vi "send_ThrottleSteeringRaw.vi"(4 "Counter":i32, 5 "200/freq":i32=1, 6 "Active":bool, 7 "CAN ID":u32=512 format="%x", 8 "Message":T2 {"APPS2" scale=0.0..4095.0; "APPS1" scale=0.0..4095.0; "Steering Angle 2" scale=0.0..4095.0; "Steering Angle 1" scale=0.0..4095.0}, 11 "CAN frame":T1[](array[typedef]) {"Data" format="%.0x"; "ArbitrationId" format="%.0x"; "Timestamp" format="%<%I:%M:%S%3u %p\n%m/%d/%Y>T"}) -> (3 "CAN frame out":T1[](array[typedef]) {"Data" format="%.0x"; "ArbitrationId" format="%.0x"; "Timestamp" format="%<%I:%M:%S%3u %p\n%m/%d/%Y>T"})   [LabVIEW 2017]
uses:
  <vilib>/nican/nican.llb/CanFrameTimed.ctl
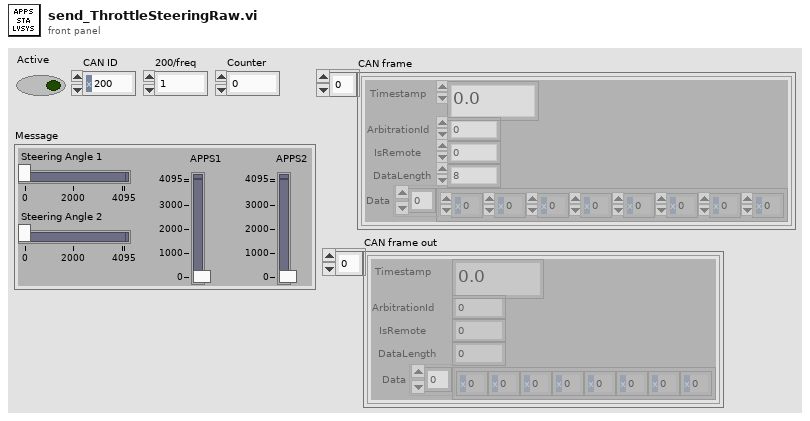
[diagram p1: front panel]
types:
  T1 = typedef "CanFrameTimed.ctl" = cluster{"Timestamp":dbl, "ArbitrationId":u32, "IsRemote":u8, "DataLength":u8, "Data":u8[]}
  T2 = cluster{"Steering Angle 1":u16, "Steering Angle 2":u16, "APPS1":u16, "APPS2":u16}
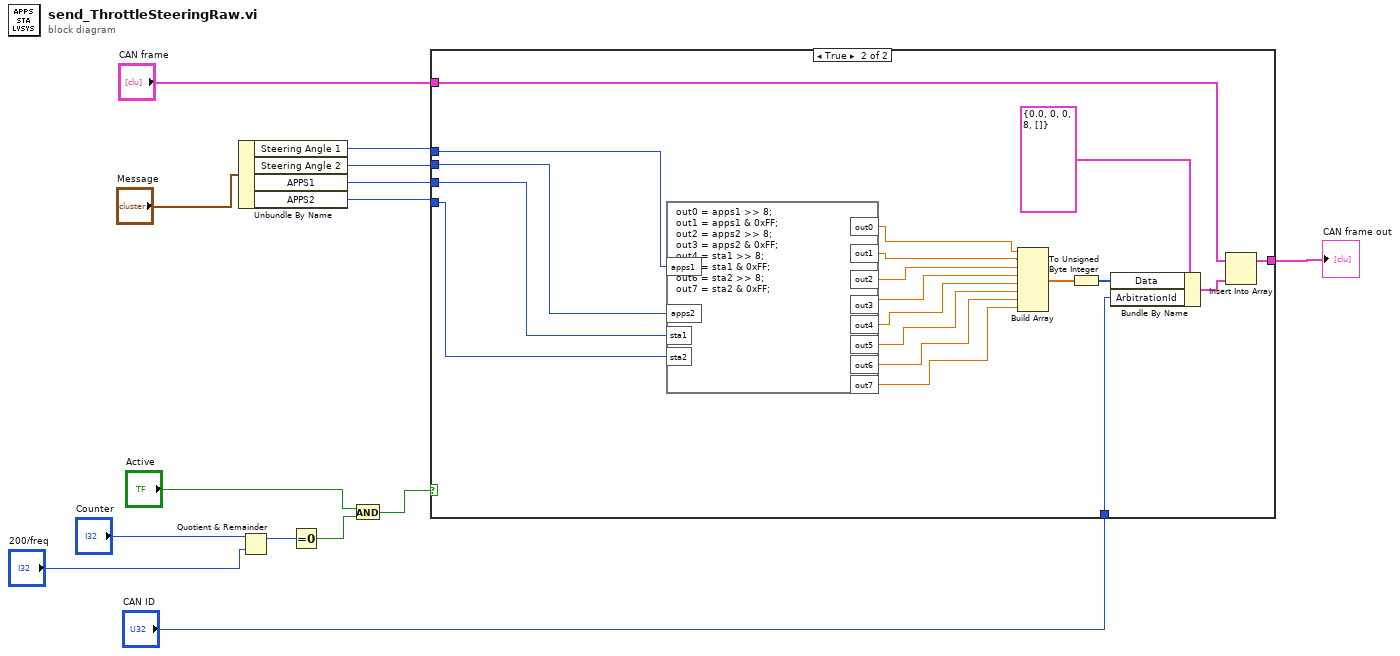
[diagram p0: block diagram]
diagram:
  n1 = Unbundle By Name("Message") -> ("Steering Angle 1"=w12:u16, "Steering Angle 2"=w13:u16, "APPS1"=w11:u16, "APPS2"=w10:u16)
  n2 = Quotient & Remainder(x="Counter", y="200/freq") -> (x-y*floor(x/y)=w5:i32)  [unwired: 1 out]
  n3 = Equal To 0?(x=w5) -> (x = 0?=w3:bool)
  n4 = And(x="Active", y=w3) -> (x .and. y?=w2:bool)
  n5 = case shown="True" w2 {
    tunnel: w13 -> [_ w18]
    tunnel: w12 -> [_ w19]
    tunnel: w11 -> [_ w17]
    tunnel: w10 -> [_ w16]
    tunnel: "CAN frame" -> [w15 w23]
    tunnel: [w15 w21] -> w8
    tunnel: "CAN ID" -> [_ w20]
    frame False {
    }
    frame True {
      n6 = formula code="out0 = apps1 >> 8;\nout1 = apps1 & 0xFF;\nout2 = apps2 >> 8;\nout3 = apps2 & 0xFF;\nout4 = sta1 >> 8;\nout5 = sta1 & 0xFF;\nout6 = sta2 >> 8;\nout7 = sta2 & 0xFF;"("apps1"=w19, "apps2"=w18, "sta1"=w17, "sta2"=w16) -> ("out1"=w33:dbl, "out2"=w32:dbl, "out3"=w31:dbl, "out0"=w34:dbl, "out4"=w30:dbl, "out5"=w29:dbl, "out6"=w28:dbl, "out7"=w27:dbl)
      n7 = Build Array(w34, w33, w32, w31, w30, w29, w28, w27) -> (w26:dbl[])
      n8 = To Unsigned Byte Integer(number=w26) -> (unsigned 8bit integer=w25:u8[])
      n9 = Bundle By Name(cluster=T1 {"Timestamp"=0.0, "ArbitrationId"=0, "IsRemote"=0, "DataLength"=8, "Data"=[]} ("CAN frame"), "Data"=w25, "ArbitrationId"=w20) -> (w22:T1)
      n10 = Insert Into Array(array=w23, new element=w22) -> (w21:T1[])  [unwired: 1 in]
    }
  }
  "CAN frame out" <- w8
